vi "AMX-电源线尾反面标签1处理函数.vi"(8 "error in (no error)":errorcluster caption="错误输入（无错误）", 9 "UI电源线正面标签1参数":T5={"Rectangle"={"Left"=0, "Top"=0, "Right"=0, "Bottom"=0, "Rotation"=0.0}, "Algorithm "=2, "Parameters"={"Number of Matches Requested"=1, "Minimum Match Score"=800.0, "Angle Ranges"=[{"Start Angle"=-180.0, "End Angle"=180.0}]}, "Advanced Options "=[{"Item"=102, "Value"=10.0}, {"Item"=106, "Value"=300.0}, {"Item"=107, "Value"=0.0}, {"Item"=108, "Value"=6.0}, {"Item"=109, "Value"=1.0}, {"Item"=114, "Value"=25.0}, {"Item"=111, "Value"=20.0}, {"Item"=112, "Value"=10.0}, {"Item"=113, "Value"=20.0}, {"Item"=103, "Value"=1.0}, {"Item"=104, "Value"=20.0}, {"Item"=105, "Value"=0.0}, {"Item"=100, "Value"=5.0}], "模板路径"=path "", "Color Plane "=0} {"Color Plane" items=["Red", "Green", "Blue", "Hue", "Saturation", "Luminance", "Value", "Intensity"]; "Advanced Options"."Item" items=["LD Sampling - Minimum Constrast"=0, "LD Sampling - Enable Subpixel Accuracy"=1, "LD Sampling - Search Strategy"=2, "LD Sampling - Subpixel Iterations"=3, "LD Sampling - Subpixel Tolerance"=4, "LD Sampling - Initial Match List Length"=5, "LD Sampling - Match List Reduction Factor"=6, "LD Sampling - Initial Step Size"=7, "LD Sampling - Intermediate Angular Accuracy"=8, "-"=9, "Pyramid - Max Pyramid Level"=100, "Pyramid - Minimum Contrast"=102, "Pyramid - Enable Subpixel Accuracy"=103, "Pyramid - Subpixel Iterations"=104, "Pyramid - Subpixel Tolerance"=105, "Pyramid - Initial Match List Length"=106, "Pyramid - Match List Reduction Factor"=107, "Pyramid - Intermediate Angular Accuracy"=108, "Pyramid - Process Border Matches"=109, "Pyramid - Min Match Separation Distance"=111, "Pyramid - Min Match Separation Angle"=112, "Pyramid - Max Match Overlap"=113, "Pyramid - Max Cache in MB"=114, "Pyramid - Clear Cache"=115, "-"=116, "Enable Defect Map"=200]; "Algorithm" items=["All", "Low Discrepancy Sampling", "Grayscale Value Pyramid", "Gradients Pyramid"]; "Rectangle"."Rotation" format="%.2f"; "Rectangle"."Left" scale=0.0..1024.0; "Rectangle"."Right" scale=0.0..1024.0}, 10 "电源线正面标签1基础参数":T3={"IsNorImage"=TRUE, "Exposure Values"=100289, "ImagePath"=path "C:/Users/hedongpo/Desktop/514-hdp/Alignment Assemble System/Test Picture/B/3.bmp"} caption="参数界面" {"Exposure Values" scale=0.0..200000.0}, 11 "Image in":T1(plugin-control)) -> (0 "error out":errorcluster caption="错误输出", 1 "Bounding Box":cluster{"x":sgl, "y":sgl}[](array[cluster]), 2 "j结果":bool, 3 "Image out":T1(plugin-control))   [LabVIEW 2017]
panel:
  out "Matches":T2(array[cluster]) {"Bounding Box"."y" format="%.2f"; "Bounding Box"."x" format="%.2f"; "Position"."y" format="%.2f"; "Position"."x" format="%.2f"; "Score" format="%.2f"; "Scale" format="%.2f"; "Angle" format="%.2f"}
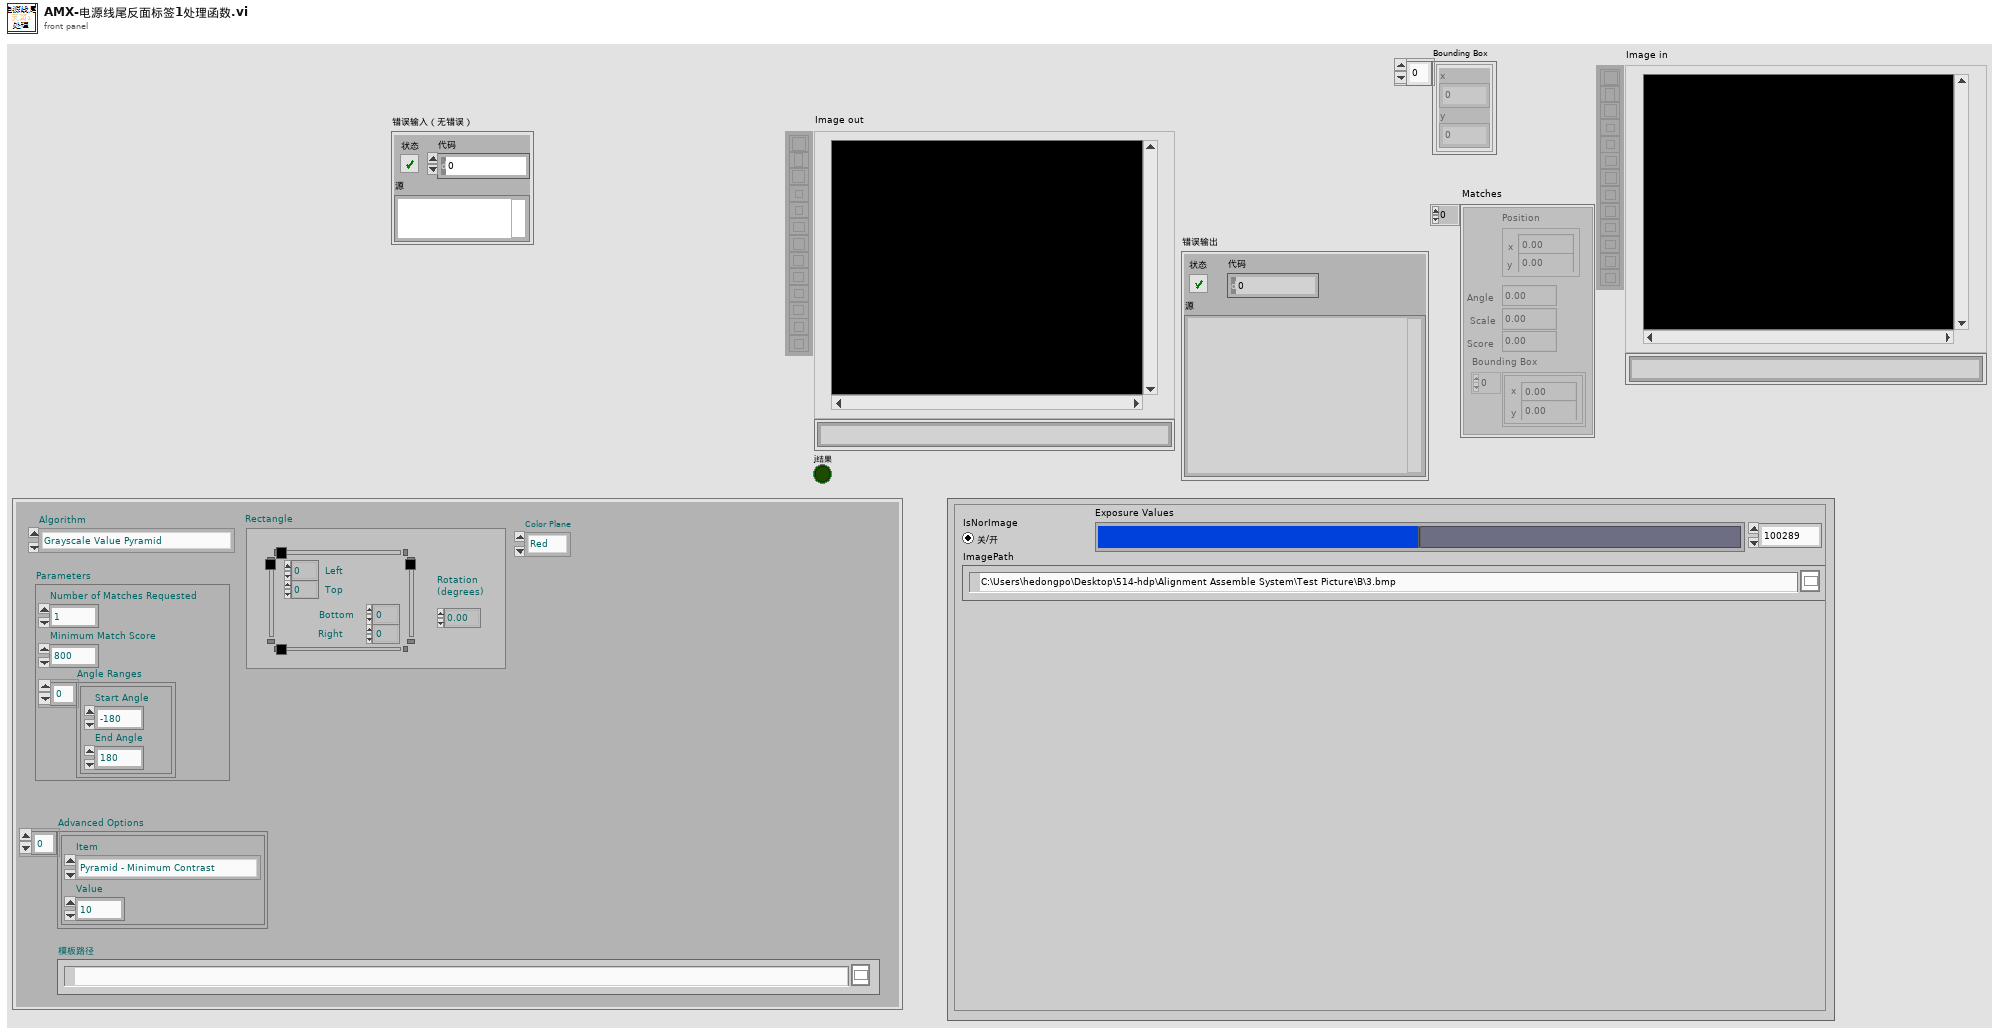
[diagram p1: front panel]
types:
  T1 = typedef "IMAQ Image.ctl" = refnum<image>
  T2 = cluster{"Position":cluster{"x":sgl, "y":sgl}, "Angle":sgl, "Scale":sgl, "Score":sgl, "Bounding Box":cluster{"x":sgl, "y":sgl}[]}[]
  T3 = cluster{"IsNorImage":bool, "Exposure Values":u32, "ImagePath":path}
  T4 = typedef "IMAQ Rectangle" = cluster{"Left":i32, "Top":i32, "Right":i32, "Bottom":i32, "Rotation":dbl}
  T5 = cluster{"Rectangle":T4, "Algorithm ":i32, "Parameters":cluster{"Number of Matches Requested":i32, "Minimum Match Score":sgl, "Angle Ranges":cluster{"Start Angle":sgl, "End Angle":sgl}[]}, "Advanced Options ":cluster{"Item":u16, "Value":dbl}[], "模板路径":path, "Color Plane ":i32}
  T6 = cluster{"Left":i32, "Top":i32, "Right":i32, "Bottom":i32}
  T7 = typedef "Image Type" = u32
  T8 = cluster{"Number of Matches Requested":i32, "Minimum Match Score":sgl, "Angle Ranges":cluster{"Start Angle":sgl, "End Angle":sgl}[]}
  T9 = typedef "ROI Descriptor" = cluster{"Global Rectangle":i32[], "Contours":cluster{"ID":enum32{"External", "Internal"}, "Type":u32, "Coordinates":i32[]}[]}
  T10 = cluster{"Position":cluster{"x":sgl, "y":sgl}, "Angle":sgl, "Scale":sgl, "Score":sgl, "Bounding Box":cluster{"x":sgl, "y":sgl}[]}
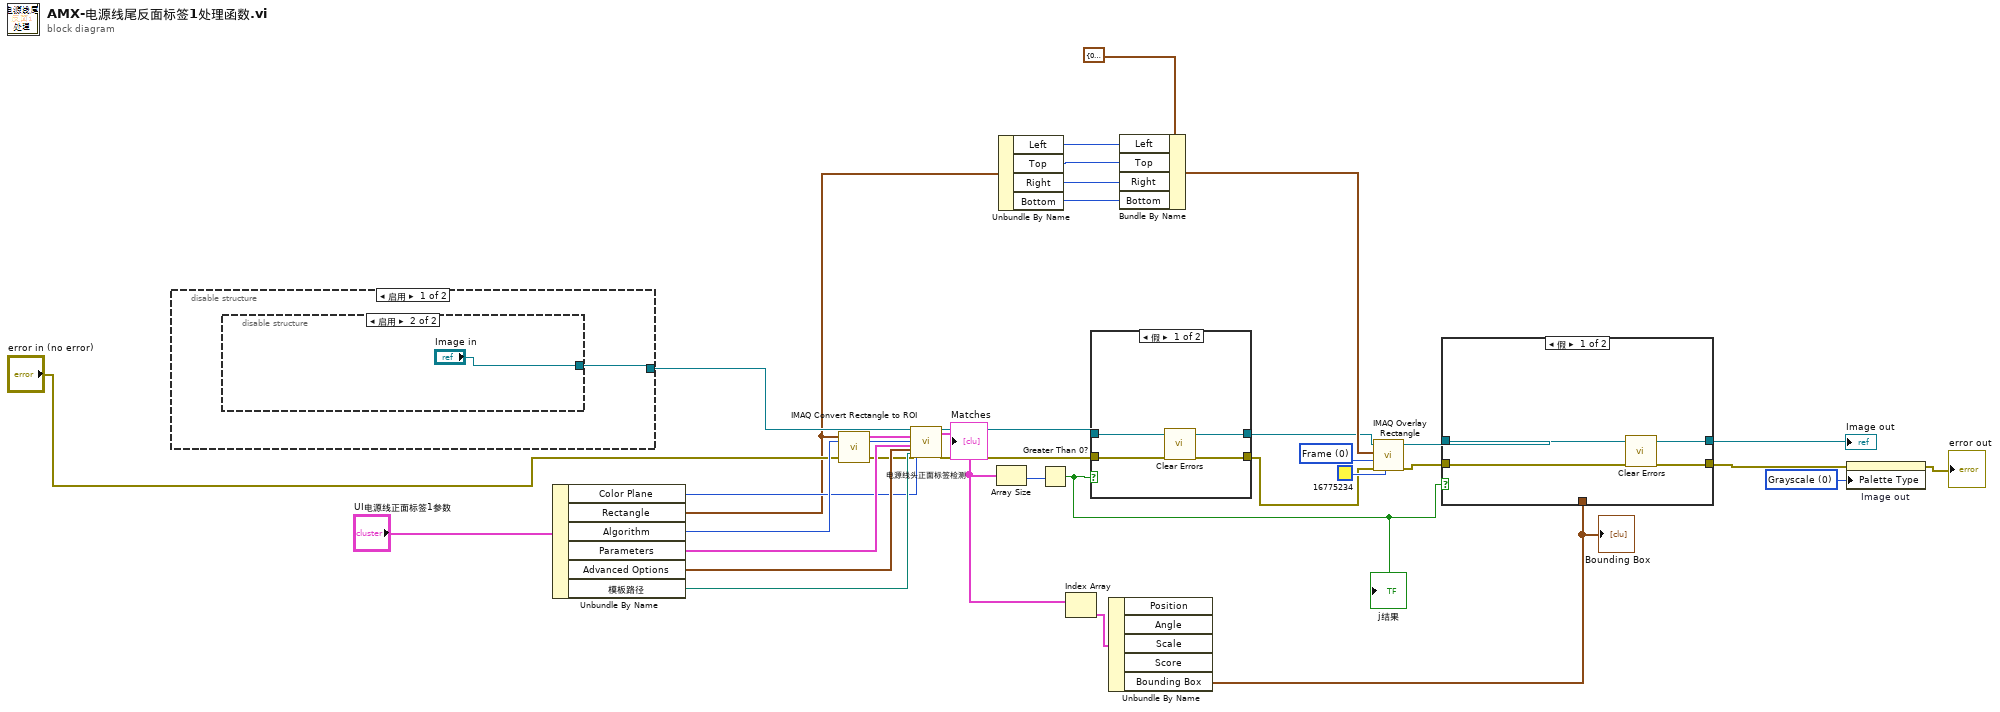
[diagram p0: block diagram]
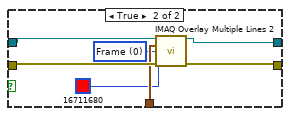
[diagram p2: hidden frame]
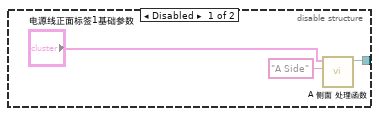
[diagram p4: hidden frame]
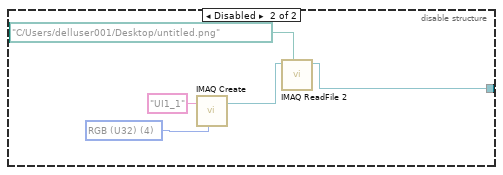
[diagram p5: hidden frame]
diagram:
  w1 = u32 0 items=["Grayscale", "Binary", "Gradient", "Rainbow", "Temperature", "User Defined", "Binary 16 Bit", "Gradient 16 Bit", "Rainbow 16 Bit", "Temperature 16 Bit", "User Defined 16 Bit"] ("Palette:Palette Type")
  w16 = u32 0 items=["Frame", "Fill", "Highlight"] ("Drawing Mode (Frame)")
  n1 = disable-structure shown="启用" {
    disable-tunnel: [w34 w39] -> w33
    frame Enabled {
      n2 = disable-structure shown="启用" {
        disable-tunnel: [w35 "Image in"] -> w34
        frame Disabled {
          n3 = call "A 侧面 处理函数.vi"("Image Name"="A Side", "ParamsUI"="电源线正面标签1基础参数") -> ("Image out"=w35:T1)  [unwired: 6 in, 3 out]
        }
        frame Enabled {
        }
      }
    }
    frame Disabled {
      w42 = T7 4 items=["Grayscale (U8)", "Grayscale (I16)", "Grayscale (SGL)", "Complex (CSG)", "RGB (U32)", "HSL (U32)", "RGB (U64)", "Grayscale (U16)"] ("Image Type")
      n4 = call "IMAQ Create"("Image Name"="UI1_1", "Image Type"=w42) -> ("New Image"=w41:T1)  [unwired: 3 in, 1 out]
      n5 = call "IMAQ ReadFile 2"("File Path"=path "C:/Users/delluser001/Desktop/untitled.png", "Image"=w41) -> ("Image Out"=w39:T1)  [unwired: 5 in, 4 out]
    }
  }
  n6 = Unbundle By Name("UI电源线正面标签1参数") -> ("Color Plane"=w25:i32, "Rectangle"=w24:T4, "Algorithm"=w31:i32, "Parameters"=w30:T8, "Advanced Options"=w29:cluster{"Item":u16, "Value":dbl}[], "模板路径"=w28:path)
  n7 = call "IMAQ Convert Rectangle to ROI"("Rectangle"=w24) -> ("ROI Descriptor"=w32:T9)  [unwired: 8 in, 1 out]
  n8 = call "电源线头正面标签检测"("Image In"=w33, "ROI Descriptor (Pattern Matching 1)"=w32, "Algorithm (Pattern Matching 1)"=w31, "Parameters (Pattern Matching 1)"=w30, "Advanced Options (Pattern Matching 1)"=w29, "Template File Path (Pattern Matching 1)"=w28, "error in"="error in (no error)", "Color Plane (Color Plane Extraction 1)"=w25) -> ("Image Out"=w11:T1, "Matches (Pattern Matching 1)"=w15:T2, "error out"=w13:errorcluster)  [unwired: 15 in, 2 out]
  "Matches" <- w15
  n9 = Array Size(array=w15) -> (size(s)=w14:i32)
  n10 = Unbundle By Name(w24) -> ("Left"=w21:i32, "Top"=w20:i32, "Right"=w19:i32, "Bottom"=w18:i32)
  n11 = Greater Than 0?(x=w14) -> (x > 0?=w6:bool)
  "j结果" <- w6
  n12 = Index Array(array=w15) -> (element=w5:T10)  [unwired: 1 in]
  n13 = case shown="假" w6 {
    tunnel: w13 -> [w46 w47]
    tunnel: [w44 w47] -> w12
    tunnel: w11 -> [w45 w48]
    tunnel: [w45 w48] -> w10
    frame False {
      n14 = call <vilib>:"Clear Errors.vi"("error in (no error)"=w46) -> ("error out"=w44:errorcluster)  [unwired: 5 in, 1 out]
    }
    frame True {
    }
  }
  n15 = Unbundle By Name(w5) -> ("Bounding Box"=w4:cluster{"x":sgl, "y":sgl}[])  [unwired: 4 out]
  "Bounding Box" <- w4
  n16 = Bundle By Name(cluster=T6 {"Left"=0, "Top"=0, "Right"=0, "Bottom"=0} ("Rectangle"), "Left"=w21, "Top"=w20, "Right"=w19, "Bottom"=w18) -> (w22:T6)
  n17 = call "IMAQ Overlay Rectangle"("Color"=u32 16775234, "error in (no error)"=w12, "Drawing Mode (Frame)"=w16, "Rectangle"=w22, "Image"=w10) -> ("error out"=w7:errorcluster, "Image Out"=w9:T1)  [unwired: 5 in]
  n18 = case shown="假" w6 {
    tunnel: w7 -> [w51 w56]
    tunnel: [w49 w55] -> w3
    tunnel: w9 -> [w50 w58]
    tunnel: [w50 w57] -> w8
    tunnel: w4 -> [_ w54]
    frame False {
      n19 = call <vilib>:"Clear Errors.vi"("error in (no error)"=w51) -> ("error out"=w49:errorcluster)  [unwired: 5 in, 1 out]
    }
    frame True {
      w53 = u32 0 items=["Frame", "Fill"] ("Drawing Mode (Frame)")
      n20 = call "IMAQ Overlay Multiple Lines 2"("Image"=w58, "Line End Points"=w54, "Drawing Mode (Frame)"=w53, "Color"=u32 16711680, "error in (no error)"=w56) -> ("Image Out"=w57:T1, "error out"=w55:errorcluster)  [unwired: 9 in]
    }
  }
  "Image out" <- w8
  n21 = property on="Image out" class="ImageControl"(error in=w3, "Palette Type"=w1) -> (error out=→"error out":errorcluster)  [unwired: 1 in, 1 out]
